vi "M9290A Measure Power.vi"(6 "Trigger Level":dbl=20.0, 7 "Route Names":string[](array[string]), 8 "error in":errorcluster, 9 "Span Frequency (50 kHz)":dbl, 10 "Center Frequency (100 MHz)":dbl=1000000000.0, 11 "VISA resource name":refnum<visa-resource-name>="ZVL") -> (0 "error out":errorcluster, 2 "Marker Amplitude (Cal)":dbl, 3 "Marker Amplitude (Raw)":dbl)   [LabVIEW 2015]
uses:
  <instrlib>/Agilent MXA Series/Public/Configure/Configure Frequency (Center Span).vi
  <instrlib>/Agilent MXA Series/Public/Configure/Trigger/Configure Trigger (Normal).vi
  <instrlib>/Agilent MXA Series/Public/Data/Read Trace (Swept SA).vi
panel:
  out "VISA resource name out":refnum<visa-resource-name>
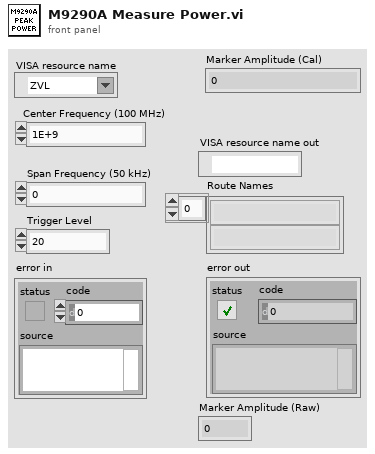
[diagram p1: front panel]
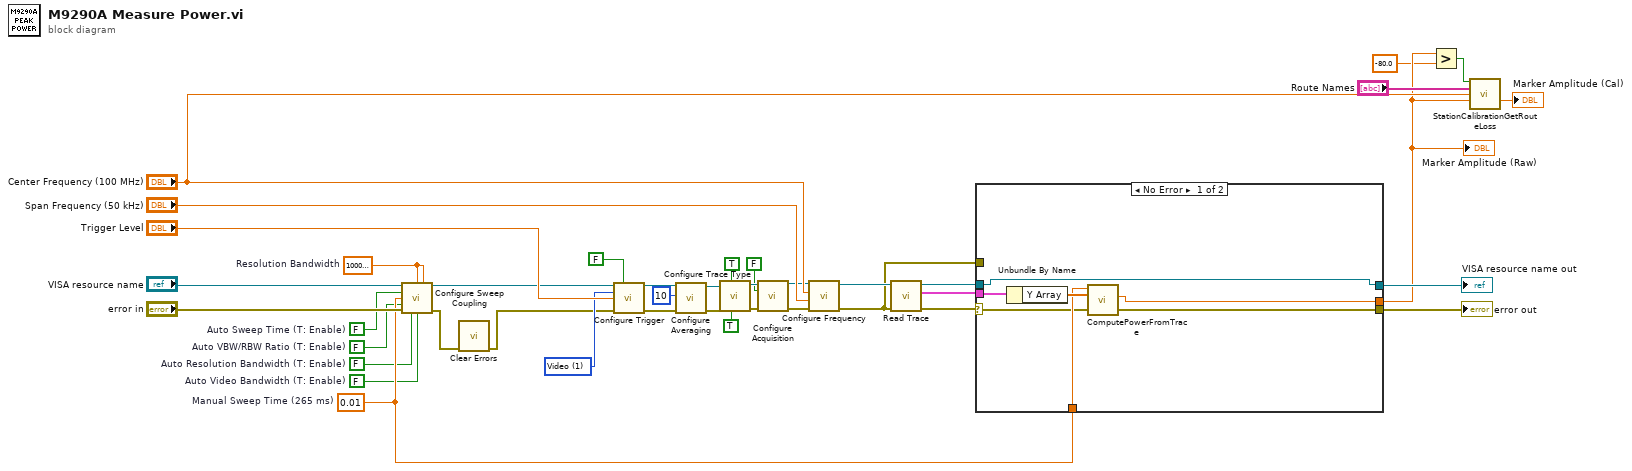
[diagram p0: block diagram]
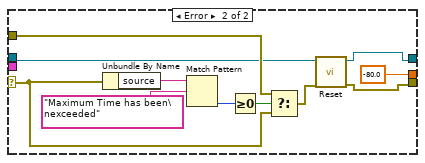
[diagram p2: hidden frame]
diagram:
  w7 = u16 1 items=["Immediate", "Video", "Line", "RF Burst", "TV", "External1", "External2"] ("Trigger Source (0: Immediate)")
  w19 = 0.01  # Manual Sweep Time (265 ms)
  w8 = FALSE  # Auto VBW/RBW Ratio (T: Enable)
  w9 = FALSE  # Auto Video Bandwidth (T: Enable)
  w12 = FALSE  # Auto Sweep Time (T: Enable)
  w11 = FALSE  # Auto Resolution Bandwidth (T: Enable)
  w10 = 1000000.0  # Resolution Bandwidth
  n1 = call <instrlib>:"Configure Sweep Coupling.vi"("VISA resource name"="VISA resource name", "Manual Resolution Bandwidth (3E+6 Hz)"=w10, "Manual Video Bandwidth (3E+6 Hz)"=w10, "Auto Sweep Time (T: Enable)"=w12, "Manual Sweep Time (0.0663 s)"=w19, "Auto VBW/RBW Ratio (T: Enable)"=w8, "error in (no error)"="error in", "Auto Resolution Bandwidth (T: Enable)"=w11, "Auto Video Bandwidth (T: Enable)"=w9) -> ("VISA resource name out"=w28:refnum<visa-resource-name>, "error out"=w2:errorcluster)  [unwired: 5 in]
  n2 = call <vilib>:"Clear Errors.vi"("error in (no error)"=w2) -> ("error out"=w1:errorcluster)  [unwired: 5 in, 1 out]
  n3 = call-poly <instrlib>:"Configure Trigger.vi"("VISA resource name"=w28, "Enable Trigger Delay (F: Disable)"=FALSE ("Enable Trigger Delay (T: Enable)"), "Trigger Source (0: Free Run)"=w7, "Trigger Level (-20 dBm)"="Trigger Level", "error in (no error)"=w1) -> ("VISA resource name out"=w16:refnum<visa-resource-name>, "error out"=w5:errorcluster)  [unwired: 9 in]
  n4 = call <instrlib>:"Configure Averaging.vi"("error in (no error)"=w5, "Average Count (100)"=10, "VISA resource name"=w16) -> ("error out"=w14:errorcluster, "VISA resource name out"=w15:refnum<visa-resource-name>)  [unwired: 7 in]
  n5 = call <instrlib>:"Configure Trace Type.vi"("Enable Trace Display (F: Disable)"=TRUE, "Enable Trace Update (F: Disable)"=TRUE, "error in (no error)"=w14, "VISA resource name"=w15) -> ("error out"=w26:errorcluster, "VISA resource name out"=w27:refnum<visa-resource-name>)  [unwired: 6 in]
  n6 = call <instrlib>:"Configure Acquisition.vi"("VISA resource name"=w27, "Enable Continuous Sweep (T: Enable)"=FALSE, "error in (no error)"=w26) -> ("VISA resource name out"=w24:refnum<visa-resource-name>, "error out"=w23:errorcluster)  [unwired: 11 in]
  n7 = call-poly <instrlib>:"Configure Frequency.vi"("error in (no error)"=w23, "Span (2.65E+10 Hz)"="Span Frequency (50 kHz)", "Center Frequency (1.325E+10 Hz)"="Center Frequency (100 MHz)", "VISA resource name"=w24) -> ("error out"=w3:errorcluster, "VISA resource name out"=w4:refnum<visa-resource-name>)  [unwired: 6 in]
  n8 = call-poly <instrlib>:"Read Trace.vi"("error in (no error)"=w3, "VISA resource name"=w4) -> ("error out"=w21:errorcluster, "Trace Waveform"=w20:cluster{"X Array":dbl[], "Y Array":dbl[]}, "VISA resource name out"=w22:refnum<visa-resource-name>)  [unwired: 7 in]
  n9 = case shown="No Error" w21 {
    selector: w21 -> [w42 w51]
    tunnel: [w42 w47] -> w40
    tunnel: [w43 w48] -> w39
    tunnel: [w41 -80.0 ("Marker Amplitude")] -> w31
    tunnel: w22 -> [w43 w49]
    tunnel: w3 -> [_ w52]
    tunnel: w20 -> [w46 _]
    tunnel: w19 -> [w44 _]
    frame No Error {
      n10 = Unbundle By Name(w46) -> ("Y Array"=w45:dbl[])
      n11 = call "ComputePowerFromTrace.vi"("Trace Array"=w45, "TraceLength"=w44) -> ("Raw Transmit Power"=w41:dbl)  [unwired: 9 in]
    }
    frame Error {
      n12 = Unbundle By Name(w51) -> ("source"=w56:string)
      n13 = Match Pattern(string=w56, regular expression="Maximum Time has been\nexceeded") -> (offset past match=w54:i32)  [unwired: 1 in, 3 out]
      n14 = Greater Or Equal To 0?(x=w54) -> (x >= 0?=w53:bool)
      n15 = Select(t=w52, s=w53, f=w51) -> (s? t:f=w50:errorcluster)
      n16 = call <instrlib>:"Reset.vi"("error in (no error)"=w50, "VISA resource name"=w49) -> ("error out"=w47:errorcluster, "VISA resource name out"=w48:refnum<visa-resource-name>)  [unwired: 8 in]
    }
  }
  "error out" <- w40
  "VISA resource name out" <- w39
  "Marker Amplitude (Raw)" <- w31
  n17 = Greater?(x=w31, y=-80.0) -> (0:w29:bool)
  n18 = call "StationCalibrationGetRouteLoss.vi"("Calibration Enabled"=w29, "Route Names"="Route Names", "Frequency"="Center Frequency (100 MHz)", "Power Level"=w31) -> ("Adjusted Power Level"=→"Marker Amplitude (Cal)":dbl)  [unwired: 8 in, 3 out]
